vi "PicoErrorString2.vi"(4 "PICO_STATUS in":T1={"status"=FALSE, "code"=0, "source"="NC"}) -> (0 "[user-defined descriptions]":string[](array[string]), 1 "String":string, 3 "[user-defined codes]":u32[](array[numeric]))   [LabVIEW 2017]
doc: "This VI takes an error cluster and if an error has occurred, displays a message box indicating the source of the error and the status code returned by the driver.\n\nThis can be used in two ways-\n1) The \"PICO_STATUS in\" (U32) cluster value will be used to search for the matching PICO_STATUS code and return a text string of the matched code. If a code is not found the string \"PICO_STATUS Unknown Error\" will be returned.\n2) Access to arrays of all PICO_STATUS codes one array of U32 enum values and the other array of matching indexed text strings with detailed describes.\nNOTE \"PICO_STATUS in\" (U32) codes have no 5000 offset unlike the \"PicoErrorString.vi\" and is designed to use with \"PicoStatus2.vi\""
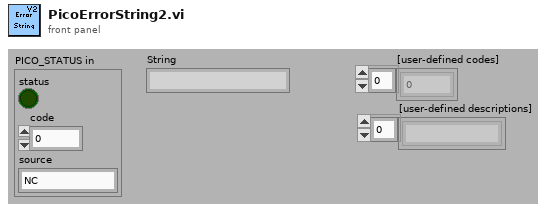
[diagram p1: front panel]
types:
  T1 = cluster{"status":bool, "code":u32, "source":string}
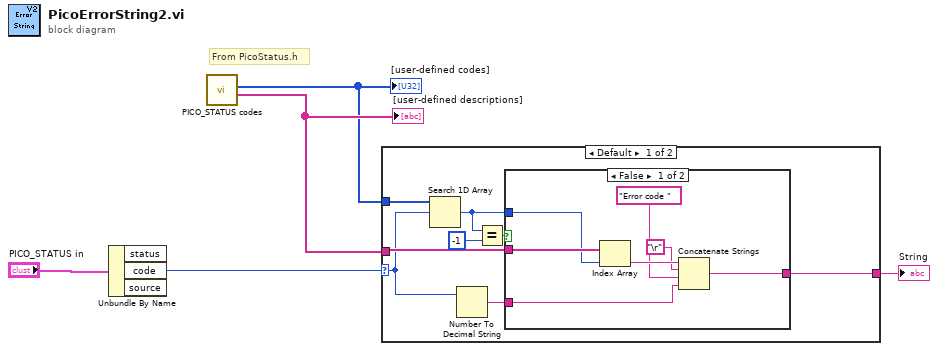
[diagram p0: block diagram]
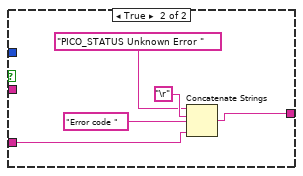
[diagram p2: hidden frame]
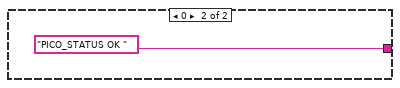
[diagram p3: hidden frame]
diagram:
  # "From PicoStatus.h"
  n1 = Unbundle By Name("PICO_STATUS in") -> ("code"=w3:u32)  [unwired: 2 out]
  n2 = call "PICO_STATUS codes.vi"() -> ("PICO_STATUS strings"=w2:string[], "PICO_STATUS codes"=w1:u32[])  [unwired: 8 in]
  "[user-defined codes]" <- w1
  "[user-defined descriptions]" <- w2
  n3 = case shown="Default" w3 {
    selector: w3 -> [w10 _]
    tunnel: w2 -> [w13 _]
    tunnel: w1 -> [w12 _]
    tunnel: [w11 "PICO_STATUS OK " ("string")] -> w5
    frame Default {
      n4 = Search 1D Array(1D array=w12, element=w10) -> (index of element=w8:i32)  [unwired: 1 in]
      n5 = Number To Decimal String(number=w10) -> (decimal integer string=w6:string)  [unwired: 1 in]
      n6 = Equal?(x=w8, y=-1) -> (x = y?=w9:bool)
      n7 = case shown="False" w9 {
        tunnel: w13 -> [w20 _]
        tunnel: w8 -> [w19 _]
        tunnel: [w17 w24] -> w11
        tunnel: w6 -> [w14 w21]
        frame False {
          n8 = Index Array(array=w20, index=w19) -> (element=w18:string)
          n9 = Concatenate Strings(w18, "\r", "Error code " ("string"), w14) -> (w17:string)
        }
        frame True {
          n10 = Concatenate Strings("PICO_STATUS Unknown Error " ("string"), "\r", "Error code " ("string"), w21) -> (w24:string)
        }
      }
    }
    frame 0 {
    }
  }
  "String" <- w5
